vi "TagDialog.vi"(8 "error in":errorcluster, 10 "new?":bool, 11 "tag":refnum<class "tag descriptor.lvclass">) -> (0 "error out":errorcluster, 1 "change?":bool, 2 "valid?":bool, 3 "new tag":refnum<class "tag descriptor.lvclass">)   [LabVIEW 2014, in "PL Framework Configuration Tool.lvlib" / "EngineTags.lvclass"]
uses:
  EngineTags.lvclass
  <vilib>/NI/Tag Bus/tag/tag descriptor.lvclass
  <vilib>/NI/Tag Bus/tag/tag descriptor.lvclass/tag descriptor.ctl
  <vilib>/NI/Tag Bus/tag/count types.vi
  <vilib>/NI/Tag Bus/tag/index to type.vi
  <vilib>/NI/Tag Bus/tag/default value polymorphs/write default value Double.vi
  <vilib>/NI/Tag Bus/tag/default value polymorphs/write default value Single.vi
  <vilib>/NI/Tag Bus/tag/default value polymorphs/write default value String.vi
  <vilib>/NI/Tag Bus/tag/default value polymorphs/write default value Boolean.vi
  <vilib>/NI/Tag Bus/tag/default value polymorphs/write default value Array of U8.vi
  <vilib>/NI/Tag Bus/tag/default value polymorphs/write default value Array of U16.vi
  <vilib>/NI/Tag Bus/tag/default value polymorphs/write default value Array of U32.vi
  <vilib>/NI/Tag Bus/tag/default value polymorphs/write default value Array of U64.vi
  <vilib>/NI/Tag Bus/tag/default value polymorphs/write default value Array of I64.vi
  <vilib>/NI/Tag Bus/tag/default value polymorphs/write default value Array of I32.vi
  <vilib>/NI/Tag Bus/tag/default value polymorphs/write default value Array of I16.vi
  <vilib>/NI/Tag Bus/tag/default value polymorphs/write default value Array of I8.vi
  <vilib>/NI/Tag Bus/tag/default value polymorphs/write default value Array of Double.vi
  <vilib>/NI/Tag Bus/tag/default value polymorphs/write default value Array of Single.vi
  <vilib>/NI/Tag Bus/tag/default value polymorphs/write default value Array of String.vi
  <vilib>/NI/Tag Bus/tag/default value polymorphs/write default value Array of Boolean.vi
  <vilib>/NI/Tag Bus/tag/default value polymorphs/write default value I64.vi
  <vilib>/NI/Tag Bus/tag/default value polymorphs/write default value I32.vi
  <vilib>/NI/Tag Bus/tag/default value polymorphs/write default value I16.vi
  <vilib>/NI/Tag Bus/tag/default value polymorphs/write default value I8.vi
  <vilib>/NI/Tag Bus/tag/default value polymorphs/write default value U64.vi
  <vilib>/NI/Tag Bus/tag/default value polymorphs/write default value U32.vi
  <vilib>/NI/Tag Bus/tag/default value polymorphs/write default value U16.vi
  <vilib>/NI/Tag Bus/tag/default value polymorphs/write default value U8.vi
  <vilib>/NI/Tag Bus/tag/default value polymorphs/read default value Double.vi
  <vilib>/NI/Tag Bus/tag/default value polymorphs/read default value Single.vi
  <vilib>/NI/Tag Bus/tag/default value polymorphs/read default value I64.vi
  <vilib>/NI/Tag Bus/tag/default value polymorphs/read default value I32.vi
  <vilib>/NI/Tag Bus/tag/default value polymorphs/read default value I16.vi
  <vilib>/NI/Tag Bus/tag/default value polymorphs/read default value I8.vi
  <vilib>/NI/Tag Bus/tag/default value polymorphs/read default value U64.vi
  <vilib>/NI/Tag Bus/tag/default value polymorphs/read default value U32.vi
  <vilib>/NI/Tag Bus/tag/default value polymorphs/read default value U16.vi
  <vilib>/NI/Tag Bus/tag/default value polymorphs/read default value U8.vi
  <vilib>/NI/Tag Bus/tag/default value polymorphs/read default value String.vi
  <vilib>/NI/Tag Bus/tag/default value polymorphs/read default value Boolean.vi
  <vilib>/NI/Tag Bus/tag/default value polymorphs/read default value Array of U8.vi
  <vilib>/NI/Tag Bus/tag/default value polymorphs/read default value Array of U16.vi
  <vilib>/NI/Tag Bus/tag/default value polymorphs/read default value Array of U32.vi
  <vilib>/NI/Tag Bus/tag/default value polymorphs/read default value Array of U64.vi
  <vilib>/NI/Tag Bus/tag/default value polymorphs/read default value Array of I64.vi
  <vilib>/NI/Tag Bus/tag/default value polymorphs/read default value Array of I32.vi
  <vilib>/NI/Tag Bus/tag/default value polymorphs/read default value Array of I16.vi
  <vilib>/NI/Tag Bus/tag/default value polymorphs/read default value Array of I8.vi
  <vilib>/NI/Tag Bus/tag/default value polymorphs/read default value Array of Double.vi
  <vilib>/NI/Tag Bus/tag/default value polymorphs/read default value Array of Single.vi
  <vilib>/NI/Tag Bus/tag/default value polymorphs/read default value Array of Boolean.vi
  <vilib>/NI/Tag Bus/tag/default value polymorphs/read default value Array of String.vi
panel:
  in  "Types":i32(listbox)
  in  "update tag":bool
  in  "Revert Button":bool
  in  "Save Button":bool
  in  "numeric type":ext caption="Default Double"
  in  "string type":string
  in  "boolean type":bool
  in  "numeric array type":ext[](array[numeric])
  in  "string array type":string[](array[string])
  in  "boolean array type":bool[](array[boolean])
  in  "Tag Name":string
  in  "Tag Description":string
  in  "Cancel Button":bool
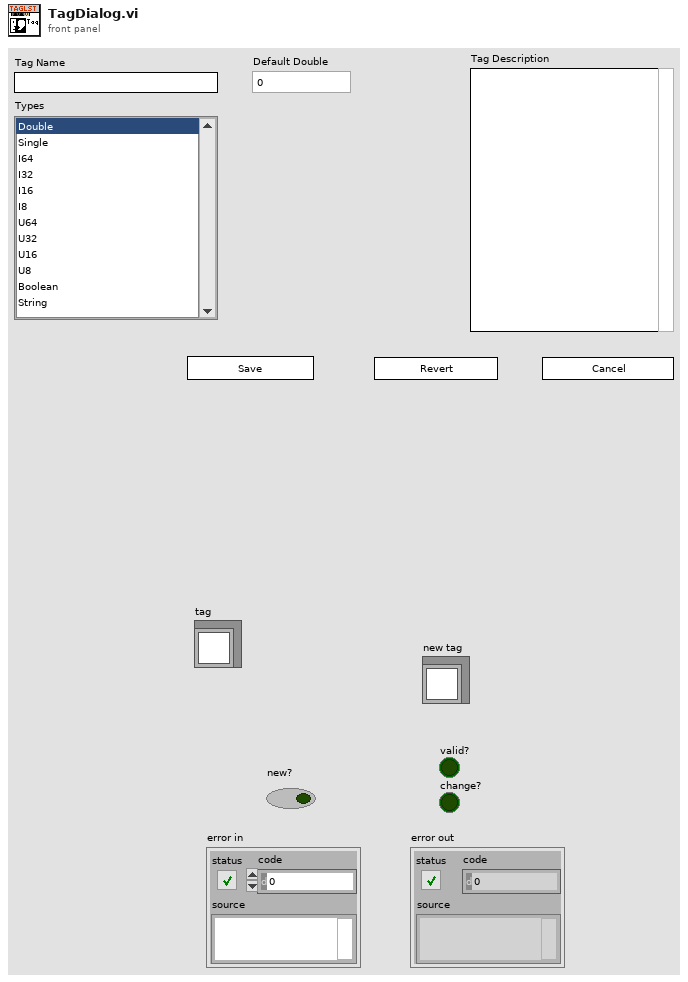
[diagram p1: front panel]
types:
  T1 = enum8{"Enabled", "Disabled", "Disabled and Grayed Out"}
  T2 = typedef "tag bus.lvlib/tag descriptor.lvclass/Data Type.ctl" = enum16{"Double", "Single", "I64", "I32", "I16", "I8", "U64", "U32", "U16", "U8", "Boolean", "String", "Array of Double", "Array of Single", "Array of I64", "Array of I32", "Array of I16", "Array of I8", "Array of U64", "Array of U32", "Array of U16", "Array of U8", "Array of Boolean", "Array of String"}
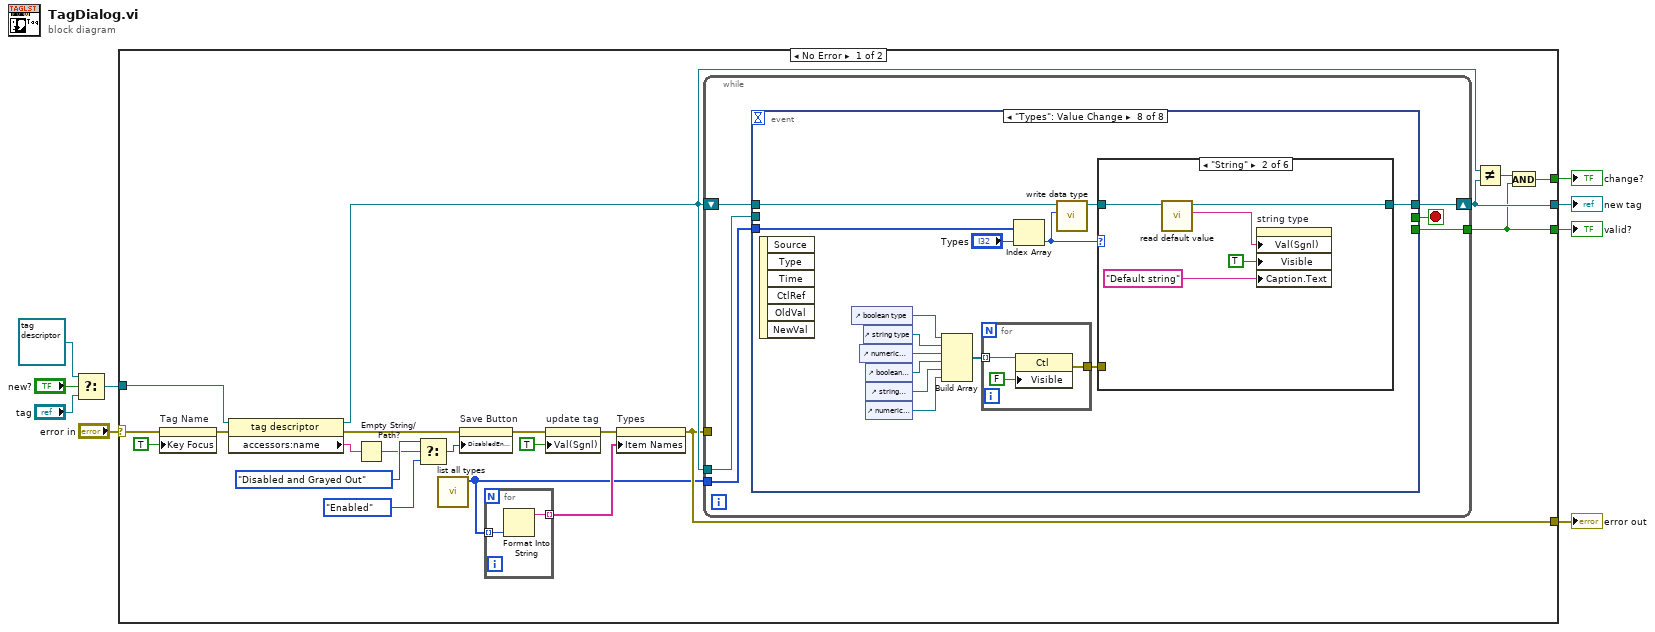
[diagram p0: block diagram]
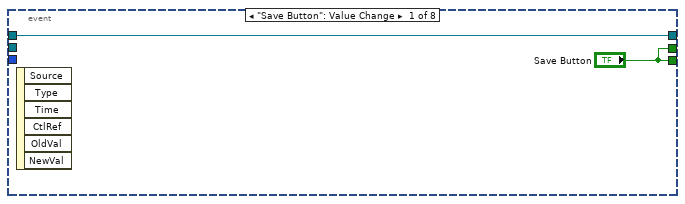
[diagram p2: hidden frame]
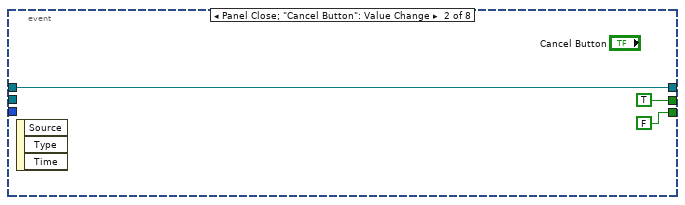
[diagram p3: hidden frame]
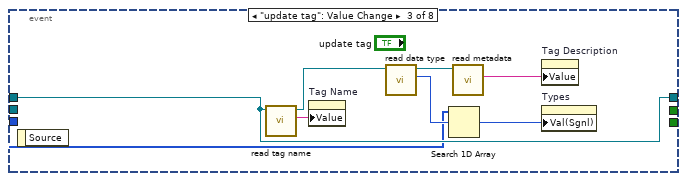
[diagram p4: hidden frame]
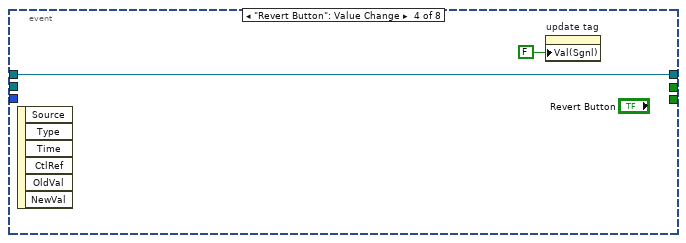
[diagram p5: hidden frame]
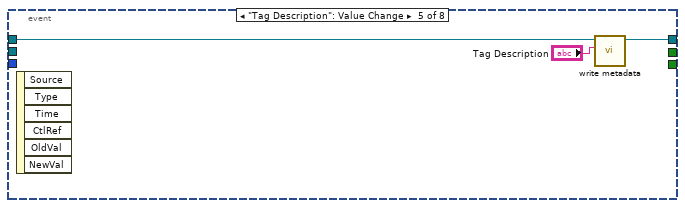
[diagram p6: hidden frame]
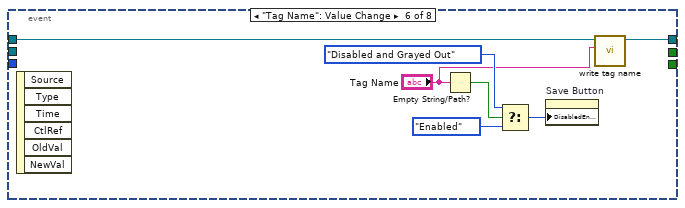
[diagram p7: hidden frame]
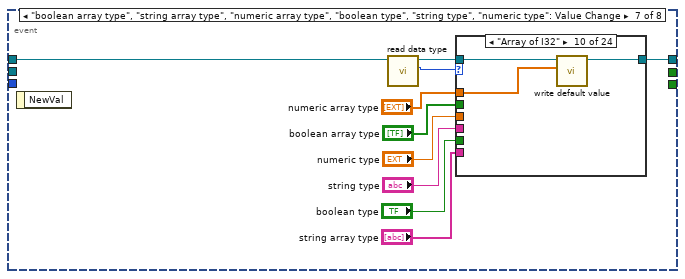
[diagram p8: hidden frame]
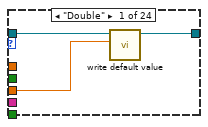
[diagram p9: hidden frame]
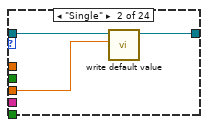
[diagram p10: hidden frame]
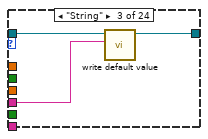
[diagram p11: hidden frame]
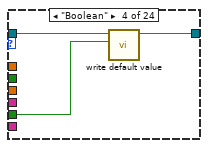
[diagram p12: hidden frame]
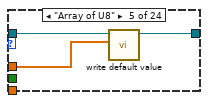
[diagram p13: hidden frame]
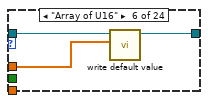
[diagram p14: hidden frame]
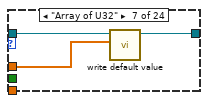
[diagram p15: hidden frame]
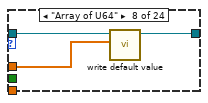
[diagram p16: hidden frame]
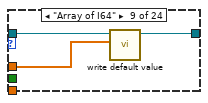
[diagram p17: hidden frame]
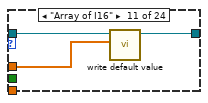
[diagram p18: hidden frame]
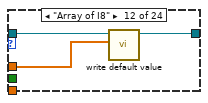
[diagram p19: hidden frame]
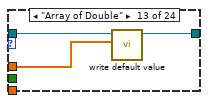
[diagram p20: hidden frame]
diagram:
  n1 = Select(t=refnum<class "tag descriptor.lvclass"> refnum ("tag"), s="new?", f="tag") -> (s? t:f=w3:refnum<class "tag descriptor.lvclass">)
  n2 = case shown="No Error" "error in" {
    selector: "error in" -> [w12 w261]
    tunnel: [w26 _] -> w9
    tunnel: [w24 _] -> w8
    tunnel: [w23 _] -> w7
    tunnel: w3 -> [w18 _]
    tunnel: [w15 w261] -> w2
    frame No Error {
      n3 = property on="Tag Name" class="Str"(error in=w12, "Key Focus"=TRUE) -> (error out=w11:errorcluster)  [unwired: 1 in, 1 out]
      n4 = property class="tag descriptor"(reference=w18, error in=w11) -> (reference out=w17:refnum<class "tag descriptor.lvclass">, error out=w21:errorcluster, "accessors:name"=w28:string)
      n5 = Empty String/Path?(string/path=w28) -> (empty?=w27:bool)
      n6 = Select(t=T1."Disabled and Grayed Out" ("Disabled"), s=w27, f=T1."Enabled") -> (s? t:f=w22:T1)
      n7 = call <vilib>:"list all types.vi"() -> ("all types"=w13:T2[])  [unwired: 11 in]
      n8 = property on="Save Button" class="Bool"(error in=w21, "DisabledEnum"=w22) -> (error out=w20:errorcluster)  [unwired: 1 in, 1 out]
      n9 = for {
        tunnel: w13 -> [w32] mode=indexing
        tunnel: [w31] -> w14 mode=indexing
        n10 = Format Into String(w32) -> (resulting string=w31:string)  [unwired: 3 in, 1 out]
      }
      n11 = property on="update tag" class="Bool (strict)"(error in=w20, "Val(Sgnl)"=TRUE ("Value (Signaling)")) -> (error out=w16:errorcluster)  [unwired: 1 in, 1 out]
      n12 = property on="Types" class="LstBox (strict)"(error in=w16, "Item Names"=w14) -> (error out=w15:errorcluster)  [unwired: 1 in, 1 out]
      n13 = while {
        tunnel: [w38] -> w23
        shift-right: [w35] -> w26
        shift-left: w17 -> [w36]
        tunnel: w17 -> [w34]
        tunnel: w15 -> [_]
        tunnel: w13 -> [w33]
        stop <- w37 stop-if-true
        n14 = event shown="[7] \"Types\": Value Change" {
          selector: _ -> [_ _ _ _ _ _ _ _]
          dyn-events: _ -> [_ _ _ _ _ _ _ _]
          timeout: _ -> [_ _ _ _ _ _ _ _]
          tunnel: ["Save Button" FALSE _ _ _ _ _ _] -> w38
          tunnel: ["Save Button" TRUE _ _ _ _ _ _] -> w37
          tunnel: w36 -> [w40 w41 w47 _ w56 w63 w65 w150]
          tunnel: [w40 w41 w47 w53 w55 w62 w64 w149] -> w35
          tunnel: w34 -> [_ _ _ w53 _ _ _ _]
          tunnel: w33 -> [_ _ w45 _ _ _ _ w148]
          event "Save Button": Value Change {
            n15 = event-data() -> ()  [unwired: 1 in, 6 out]
          }
          event Panel Close; "Cancel Button": Value Change {
            n16 = event-data() -> ()  [unwired: 1 in, 3 out]
          }
          event "update tag": Value Change {
            n17 = event-data() -> ()  [unwired: 1 in, 1 out]
            n18 = call <vilib>:"read tag name.vi"("system tag in"=w47) -> ("name"=w51:string, "system tag out"=w50:refnum<class "tag descriptor.lvclass">)  [unwired: 8 in, 1 out]
            n19 = property on="Tag Name" class="Str"("Value"=w51) -> ()  [unwired: 2 in, 2 out]
            n20 = call <vilib>:"read data type.vi"("system tag in"=w50) -> ("data type"=w46:T2, "system tag out"=w48:refnum<class "tag descriptor.lvclass">)  [unwired: 8 in, 1 out]
            n21 = Search 1D Array(1D array=w45, element=w46) -> (index of element=w44:i32)  [unwired: 1 in]
            n22 = call <vilib>:"read metadata.vi"("system tag in"=w48) -> ("metadata"=w49:string)  [unwired: 8 in, 2 out]
            n23 = property on="Tag Description" class="Str"("Value"=w49) -> ()  [unwired: 2 in, 2 out]
            n24 = property on="Types" class="LstBox (strict)"("Val(Sgnl)"=w44) -> ()  [unwired: 2 in, 2 out]
          }
          event "Revert Button": Value Change {
            n25 = event-data() -> ()  [unwired: 1 in, 6 out]
            n26 = property on="update tag" class="Bool (strict)"("Val(Sgnl)"=FALSE ("Value (Signaling)")) -> ()  [unwired: 2 in, 2 out]
          }
          event "Tag Description": Value Change {
            n27 = event-data() -> ()  [unwired: 1 in, 6 out]
            n28 = call <vilib>:"write metadata.vi"("metadata"="Tag Description", "system tag in"=w56) -> ("system tag out"=w55:refnum<class "tag descriptor.lvclass">)  [unwired: 8 in, 1 out]
          }
          event "Tag Name": Value Change {
            n29 = event-data() -> ()  [unwired: 1 in, 6 out]
            n30 = Empty String/Path?(string/path="Tag Name") -> (empty?=w59:bool)
            n31 = Select(t=T1."Disabled and Grayed Out" ("Disabled"), s=w59, f=T1."Enabled") -> (s? t:f=w58:T1)
            n32 = property on="Save Button" class="Bool"("DisabledEnum"=w58) -> ()  [unwired: 2 in, 2 out]
            n33 = call <vilib>:"write tag name.vi"("name"="Tag Name", "system tag in"=w63) -> ("system tag out"=w62:refnum<class "tag descriptor.lvclass">)  [unwired: 8 in, 1 out]
          }
          event "boolean array type", "string array type", "numeric array type", "boolean type", "string type", "numeric type": Value Change {
            n34 = event-data() -> ()  [unwired: 1 in, 1 out]
            n35 = call <vilib>:"read data type.vi"("system tag in"=w65) -> ("data type"=w66:T2, "system tag out"=w67:refnum<class "tag descriptor.lvclass">)  [unwired: 8 in, 1 out]
            n36 = case shown="\"Array of I32\"" w66 {
              tunnel: [w76 w79 w82 w85 w88 w91 w94 w97 w100 w103 w106 w109 w112 w115 w118 w121 w124 w127 w130 w133 w136 w139 w142 w145] -> w64
              tunnel: w67 -> [w75 w78 w81 w84 w87 w90 w93 w96 w99 w102 w105 w108 w111 w114 w117 w120 w123 w126 w129 w132 w135 w138 w141 w144]
              tunnel: "numeric type" -> [w74 w77 _ _ _ _ _ _ _ _ _ _ _ _ _ _ w122 w125 w128 w131 w134 w137 w140 w143]
              tunnel: "string type" -> [_ _ w80 _ _ _ _ _ _ _ _ _ _ _ _ _ _ _ _ _ _ _ _ _]
              tunnel: "boolean type" -> [_ _ _ w83 _ _ _ _ _ _ _ _ _ _ _ _ _ _ _ _ _ _ _ _]
              tunnel: "numeric array type" -> [_ _ _ _ w86 w89 w92 w95 w98 w101 w104 w107 w110 w113 _ _ _ _ _ _ _ _ _ _]
              tunnel: "string array type" -> [_ _ _ _ _ _ _ _ _ _ _ _ _ _ w116 _ _ _ _ _ _ _ _ _]
              tunnel: "boolean array type" -> [_ _ _ _ _ _ _ _ _ _ _ _ _ _ _ w119 _ _ _ _ _ _ _ _]
              frame "Double" {
                n37 = call-poly <vilib>:"write default value.vi"("default value"=w74, "system tag in"=w75) -> ("system tag out"=w76:refnum<class "tag descriptor.lvclass">)  [unwired: 8 in, 1 out]
              }
              frame "Single" {
                n38 = call-poly <vilib>:"write default value.vi"("default value"=w77, "system tag in"=w78) -> ("system tag out"=w79:refnum<class "tag descriptor.lvclass">)  [unwired: 8 in, 1 out]
              }
              frame "String" {
                n39 = call-poly <vilib>:"write default value.vi"("default value"=w80, "system tag in"=w81) -> ("system tag out"=w82:refnum<class "tag descriptor.lvclass">)  [unwired: 8 in, 1 out]
              }
              frame "Boolean" {
                n40 = call-poly <vilib>:"write default value.vi"("default value"=w83, "system tag in"=w84) -> ("system tag out"=w85:refnum<class "tag descriptor.lvclass">)  [unwired: 8 in, 1 out]
              }
              frame "Array of U8" {
                n41 = call-poly <vilib>:"write default value.vi"("default value"=w86, "system tag in"=w87) -> ("system tag out"=w88:refnum<class "tag descriptor.lvclass">)  [unwired: 8 in, 1 out]
              }
              frame "Array of U16" {
                n42 = call-poly <vilib>:"write default value.vi"("default value"=w89, "system tag in"=w90) -> ("system tag out"=w91:refnum<class "tag descriptor.lvclass">)  [unwired: 8 in, 1 out]
              }
              frame "Array of U32" {
                n43 = call-poly <vilib>:"write default value.vi"("default value"=w92, "system tag in"=w93) -> ("system tag out"=w94:refnum<class "tag descriptor.lvclass">)  [unwired: 8 in, 1 out]
              }
              frame "Array of U64" {
                n44 = call-poly <vilib>:"write default value.vi"("default value"=w95, "system tag in"=w96) -> ("system tag out"=w97:refnum<class "tag descriptor.lvclass">)  [unwired: 8 in, 1 out]
              }
              frame "Array of I64" {
                n45 = call-poly <vilib>:"write default value.vi"("default value"=w98, "system tag in"=w99) -> ("system tag out"=w100:refnum<class "tag descriptor.lvclass">)  [unwired: 8 in, 1 out]
              }
              frame "Array of I32" {
                n46 = call-poly <vilib>:"write default value.vi"("default value"=w101, "system tag in"=w102) -> ("system tag out"=w103:refnum<class "tag descriptor.lvclass">)  [unwired: 8 in, 1 out]
              }
              frame "Array of I16" {
                n47 = call-poly <vilib>:"write default value.vi"("default value"=w104, "system tag in"=w105) -> ("system tag out"=w106:refnum<class "tag descriptor.lvclass">)  [unwired: 8 in, 1 out]
              }
              frame "Array of I8" {
                n48 = call-poly <vilib>:"write default value.vi"("default value"=w107, "system tag in"=w108) -> ("system tag out"=w109:refnum<class "tag descriptor.lvclass">)  [unwired: 8 in, 1 out]
              }
              frame "Array of Double" {
                n49 = call-poly <vilib>:"write default value.vi"("default value"=w110, "system tag in"=w111) -> ("system tag out"=w112:refnum<class "tag descriptor.lvclass">)  [unwired: 8 in, 1 out]
              }
              frame "Array of Single" {
                n50 = call-poly <vilib>:"write default value.vi"("default value"=w113, "system tag in"=w114) -> ("system tag out"=w115:refnum<class "tag descriptor.lvclass">)  [unwired: 8 in, 1 out]
              }
              frame "Array of String" {
                n51 = call-poly <vilib>:"write default value.vi"("default value"=w116, "system tag in"=w117) -> ("system tag out"=w118:refnum<class "tag descriptor.lvclass">)  [unwired: 8 in, 1 out]
              }
              frame "Array of Boolean" {
                n52 = call-poly <vilib>:"write default value.vi"("default value"=w119, "system tag in"=w120) -> ("system tag out"=w121:refnum<class "tag descriptor.lvclass">)  [unwired: 8 in, 1 out]
              }
              frame "I64" {
                n53 = call-poly <vilib>:"write default value.vi"("default value"=w122, "system tag in"=w123) -> ("system tag out"=w124:refnum<class "tag descriptor.lvclass">)  [unwired: 8 in, 1 out]
              }
              frame "I32" {
                n54 = call-poly <vilib>:"write default value.vi"("default value"=w125, "system tag in"=w126) -> ("system tag out"=w127:refnum<class "tag descriptor.lvclass">)  [unwired: 8 in, 1 out]
              }
              frame "I16" {
                n55 = call-poly <vilib>:"write default value.vi"("default value"=w128, "system tag in"=w129) -> ("system tag out"=w130:refnum<class "tag descriptor.lvclass">)  [unwired: 8 in, 1 out]
              }
              frame "I8" {
                n56 = call-poly <vilib>:"write default value.vi"("default value"=w131, "system tag in"=w132) -> ("system tag out"=w133:refnum<class "tag descriptor.lvclass">)  [unwired: 8 in, 1 out]
              }
              frame "U64" {
                n57 = call-poly <vilib>:"write default value.vi"("default value"=w134, "system tag in"=w135) -> ("system tag out"=w136:refnum<class "tag descriptor.lvclass">)  [unwired: 8 in, 1 out]
              }
              frame "U32" {
                n58 = call-poly <vilib>:"write default value.vi"("default value"=w137, "system tag in"=w138) -> ("system tag out"=w139:refnum<class "tag descriptor.lvclass">)  [unwired: 8 in, 1 out]
              }
              frame "U16" {
                n59 = call-poly <vilib>:"write default value.vi"("default value"=w140, "system tag in"=w141) -> ("system tag out"=w142:refnum<class "tag descriptor.lvclass">)  [unwired: 8 in, 1 out]
              }
              frame "U8" {
                n60 = call-poly <vilib>:"write default value.vi"("default value"=w143, "system tag in"=w144) -> ("system tag out"=w145:refnum<class "tag descriptor.lvclass">)  [unwired: 8 in, 1 out]
              }
            }
          }
          event "Types": Value Change {
            n61 = event-data() -> ()  [unwired: 1 in, 6 out]
            n62 = control-ref of="boolean type"() -> (w159:refnum<vi>)
            n63 = control-ref of="numeric type"() -> (w157:refnum<vi>)
            n64 = control-ref of="string type"() -> (w158:refnum<vi>)
            n65 = control-ref of="boolean array type"() -> (w156:refnum<vi>)
            n66 = control-ref of="string array type"() -> (w155:refnum<vi>)
            n67 = control-ref of="numeric array type"() -> (w154:refnum<vi>)
            n68 = Build Array(w159, w158, w157, w156, w155, w154) -> (w153:refnum<vi>[])
            n69 = for {
              tunnel: w153 -> [w260] mode=indexing
              tunnel: [w258] -> w151
              n70 = property class="Ctl"(reference=w260, "Visible"=FALSE) -> (error out=w258:errorcluster)  [unwired: 1 in, 1 out]
            }
            n71 = Index Array(array=w148, index="Types") -> (element=w146:T2)
            n72 = call <vilib>:"write data type.vi"("data type"=w146, "system tag in"=w150) -> ("system tag out"=w152:refnum<class "tag descriptor.lvclass">)  [unwired: 8 in, 1 out]
            n73 = case shown="\"String\"" w146 {
              selector: w146 -> [w160 _ _ w209 _ _]
              tunnel: w152 -> [w163 w201 w206 w212 w250 w255]
              tunnel: [w162 w200 w205 w211 w249 w253] -> w149
              tunnel: w151 -> [_ _ _ _ _ _]
              frame "Double".."U8" {
                n74 = case shown="\"I64\"" w160 {
                  tunnel: w163 -> [w168 w171 w174 w177 w180 w183 w186 w189 w192 w195 w198]
                  tunnel: [w168 w170 w173 w176 w179 w182 w185 w188 w191 w194 w197] -> w162
                  tunnel: [ext 0.0 ("default value") w169 w172 w175 w178 w181 w184 w187 w190 w193 w196] -> w161
                  frame Default {
                  }
                  frame "Double" {
                    n75 = call-poly <vilib>:"read default value.vi"("system tag in"=w171) -> ("default value"=w169:dbl, "system tag out"=w170:refnum<class "tag descriptor.lvclass">)  [unwired: 7 in, 2 out]
                  }
                  frame "Single" {
                    n76 = call-poly <vilib>:"read default value.vi"("system tag in"=w174) -> ("default value"=w172:sgl, "system tag out"=w173:refnum<class "tag descriptor.lvclass">)  [unwired: 7 in, 2 out]
                  }
                  frame "I64" {
                    n77 = call-poly <vilib>:"read default value.vi"("system tag in"=w177) -> ("default value"=w175:i64, "system tag out"=w176:refnum<class "tag descriptor.lvclass">)  [unwired: 7 in, 2 out]
                  }
                  frame "I32" {
                    n78 = call-poly <vilib>:"read default value.vi"("system tag in"=w180) -> ("default value"=w178:i32, "system tag out"=w179:refnum<class "tag descriptor.lvclass">)  [unwired: 7 in, 2 out]
                  }
                  frame "I16" {
                    n79 = call-poly <vilib>:"read default value.vi"("system tag in"=w183) -> ("default value"=w181:i16, "system tag out"=w182:refnum<class "tag descriptor.lvclass">)  [unwired: 7 in, 2 out]
                  }
                  frame "I8" {
                    n80 = call-poly <vilib>:"read default value.vi"("system tag in"=w186) -> ("default value"=w184:i8, "system tag out"=w185:refnum<class "tag descriptor.lvclass">)  [unwired: 7 in, 2 out]
                  }
                  frame "U64" {
                    n81 = call-poly <vilib>:"read default value.vi"("system tag in"=w189) -> ("default value"=w187:u64, "system tag out"=w188:refnum<class "tag descriptor.lvclass">)  [unwired: 7 in, 2 out]
                  }
                  frame "U32" {
                    n82 = call-poly <vilib>:"read default value.vi"("system tag in"=w192) -> ("default value"=w190:u32, "system tag out"=w191:refnum<class "tag descriptor.lvclass">)  [unwired: 7 in, 2 out]
                  }
                  frame "U16" {
                    n83 = call-poly <vilib>:"read default value.vi"("system tag in"=w195) -> ("default value"=w193:u16, "system tag out"=w194:refnum<class "tag descriptor.lvclass">)  [unwired: 7 in, 2 out]
                  }
                  frame "U8" {
                    n84 = call-poly <vilib>:"read default value.vi"("system tag in"=w198) -> ("default value"=w196:u8, "system tag out"=w197:refnum<class "tag descriptor.lvclass">)  [unwired: 7 in, 2 out]
                  }
                }
                n85 = Format Into String(format string="Default %s", w160) -> (resulting string=w165:string)  [unwired: 2 in, 1 out]
                n86 = property on="numeric type" class="DigNum (strict)"("Val(Sgnl)"=w161, "Visible"=TRUE, "Caption.Text"=w165) -> ()  [unwired: 2 in, 2 out]
              }
              frame "String" {
                n87 = call-poly <vilib>:"read default value.vi"("system tag in"=w201) -> ("default value"=w199:string, "system tag out"=w200:refnum<class "tag descriptor.lvclass">)  [unwired: 7 in, 2 out]
                n88 = property on="string type" class="Str"("Val(Sgnl)"=w199, "Visible"=TRUE, "Caption.Text"="Default string" ("format string")) -> ()  [unwired: 2 in, 2 out]
              }
              frame "Boolean" {
                n89 = call-poly <vilib>:"read default value.vi"("system tag in"=w206) -> ("default value"=w204:bool, "system tag out"=w205:refnum<class "tag descriptor.lvclass">)  [unwired: 7 in, 2 out]
                n90 = property on="boolean type" class="Bool (strict)"("Val(Sgnl)"=w204, "Visible"=TRUE, "Caption.Text"="Default booleans" ("format string")) -> ()  [unwired: 2 in, 2 out]
              }
              frame "Array of Double".."Array of U8" {
                n91 = case shown="\"Array of U8\"" w209 {
                  tunnel: w212 -> [w217 w220 w223 w226 w229 w232 w235 w238 w241 w244 w247]
                  tunnel: [w217 w219 w222 w225 w228 w231 w234 w237 w240 w243 w246] -> w211
                  tunnel: [ext[] [] ("default value") w218 w221 w224 w227 w230 w233 w236 w239 w242 w245] -> w210
                  frame Default {
                  }
                  frame "Array of U8" {
                    n92 = call-poly <vilib>:"read default value.vi"("system tag in"=w220) -> ("default value"=w218:u8[], "system tag out"=w219:refnum<class "tag descriptor.lvclass">)  [unwired: 7 in, 2 out]
                  }
                  frame "Array of U16" {
                    n93 = call-poly <vilib>:"read default value.vi"("system tag in"=w223) -> ("default value"=w221:u16[], "system tag out"=w222:refnum<class "tag descriptor.lvclass">)  [unwired: 7 in, 2 out]
                  }
                  frame "Array of U32" {
                    n94 = call-poly <vilib>:"read default value.vi"("system tag in"=w226) -> ("default value"=w224:u32[], "system tag out"=w225:refnum<class "tag descriptor.lvclass">)  [unwired: 7 in, 2 out]
                  }
                  frame "Array of U64" {
                    n95 = call-poly <vilib>:"read default value.vi"("system tag in"=w229) -> ("default value"=w227:u64[], "system tag out"=w228:refnum<class "tag descriptor.lvclass">)  [unwired: 7 in, 2 out]
                  }
                  frame "Array of I64" {
                    n96 = call-poly <vilib>:"read default value.vi"("system tag in"=w232) -> ("default value"=w230:i64[], "system tag out"=w231:refnum<class "tag descriptor.lvclass">)  [unwired: 7 in, 2 out]
                  }
                  frame "Array of I32" {
                    n97 = call-poly <vilib>:"read default value.vi"("system tag in"=w235) -> ("default value"=w233:i32[], "system tag out"=w234:refnum<class "tag descriptor.lvclass">)  [unwired: 7 in, 2 out]
                  }
                  frame "Array of I16" {
                    n98 = call-poly <vilib>:"read default value.vi"("system tag in"=w238) -> ("default value"=w236:i16[], "system tag out"=w237:refnum<class "tag descriptor.lvclass">)  [unwired: 7 in, 2 out]
                  }
                  frame "Array of I8" {
                    n99 = call-poly <vilib>:"read default value.vi"("system tag in"=w241) -> ("default value"=w239:i8[], "system tag out"=w240:refnum<class "tag descriptor.lvclass">)  [unwired: 7 in, 2 out]
                  }
                  frame "Array of Double" {
                    n100 = call-poly <vilib>:"read default value.vi"("system tag in"=w244) -> ("default value"=w242:dbl[], "system tag out"=w243:refnum<class "tag descriptor.lvclass">)  [unwired: 7 in, 2 out]
                  }
                  frame "Array of Single" {
                    n101 = call-poly <vilib>:"read default value.vi"("system tag in"=w247) -> ("default value"=w245:sgl[], "system tag out"=w246:refnum<class "tag descriptor.lvclass">)  [unwired: 7 in, 2 out]
                  }
                }
                n102 = Format Into String(format string="Default %ss", w209) -> (resulting string=w214:string)  [unwired: 2 in, 1 out]
                n103 = property on="numeric array type" class="Arr (strict)"("Val(Sgnl)"=w210, "Visible"=TRUE, "Caption.Text"=w214) -> ()  [unwired: 2 in, 2 out]
              }
              frame "Array of Boolean" {
                n104 = call-poly <vilib>:"read default value.vi"("system tag in"=w250) -> ("default value"=w248:bool[], "system tag out"=w249:refnum<class "tag descriptor.lvclass">)  [unwired: 7 in, 2 out]
                n105 = property on="boolean array type" class="Arr (strict)"("Val(Sgnl)"=w248, "Visible"=TRUE, "Caption.Text"="Default booleans") -> ()  [unwired: 2 in, 2 out]
              }
              frame "Array of String" {
                n106 = call-poly <vilib>:"read default value.vi"("system tag in"=w255) -> ("default value"=w254:string[], "system tag out"=w253:refnum<class "tag descriptor.lvclass">)  [unwired: 7 in, 2 out]
                n107 = property on="string array type" class="Arr (strict)"("Val(Sgnl)"=w254, "Visible"=TRUE, "Caption.Text"="Default strings") -> ()  [unwired: 2 in, 2 out]
              }
            }
          }
        }
      }
      n108 = Not Equal?(x=w17, y=w26) -> (x != y?=w25:bool)
      n109 = And(x=w25, y=w23) -> (x .and. y?=w24:bool)
    }
    frame Error {
    }
  }
  "error out" <- w2
  "valid?" <- w7
  "change?" <- w8
  "new tag" <- w9
